vi "Liblinear - Scale Problem Linear.vi"(8 "error in (no error)":errorcluster, 10 "X Scaling limits":cluster{"X lower":dbl, "X upper":dbl}={"X lower"=0.0, "X upper"=1.0}, 11 "Problem":T1={"y"=[], "x"=[], "bias"=-1.0}) -> (0 "error out":errorcluster, 2 "xmaxmin":cluster{"min":dbl, "max":dbl}[](array[cluster]), 3 "Scaled problem":T1={"y"=[], "x"=[], "bias"=-1.0})   [LabVIEW 2015]
doc: "Scales the problem similarly to the svm-scale tool bundled with libsvm.\nAlways use the output from this VI to scale the test set instead of scaling individually."
uses:
  Liblinear/Controls/liblinear_problem.ctl
  LibSVM Sparse/Wrapper API/Controls/svm_node.ctl
  Controls/Statemachine_ScaleProblem.ctl
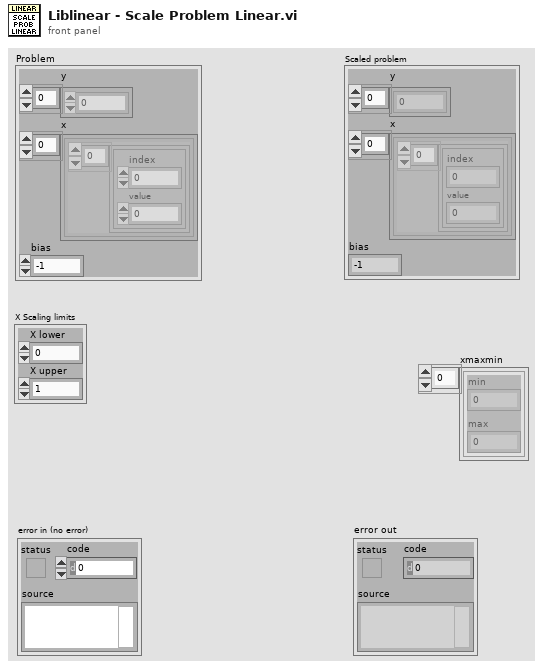
[diagram p1: front panel]
types:
  T1 = typedef "liblinear_problem.ctl" = cluster{"y":dbl[], "x":cluster{T2[]}[], "bias":dbl}
  T2 = typedef "svm_node.ctl" = cluster{"index":i32, "value":dbl}
  T3 = typedef "Statemachine_ScaleProblem.ctl" = enum16{"Input verification: Limits", "Input verification: Ascending indices", "Find max/min index", "Find max/min features", "Scale", "Stop"}
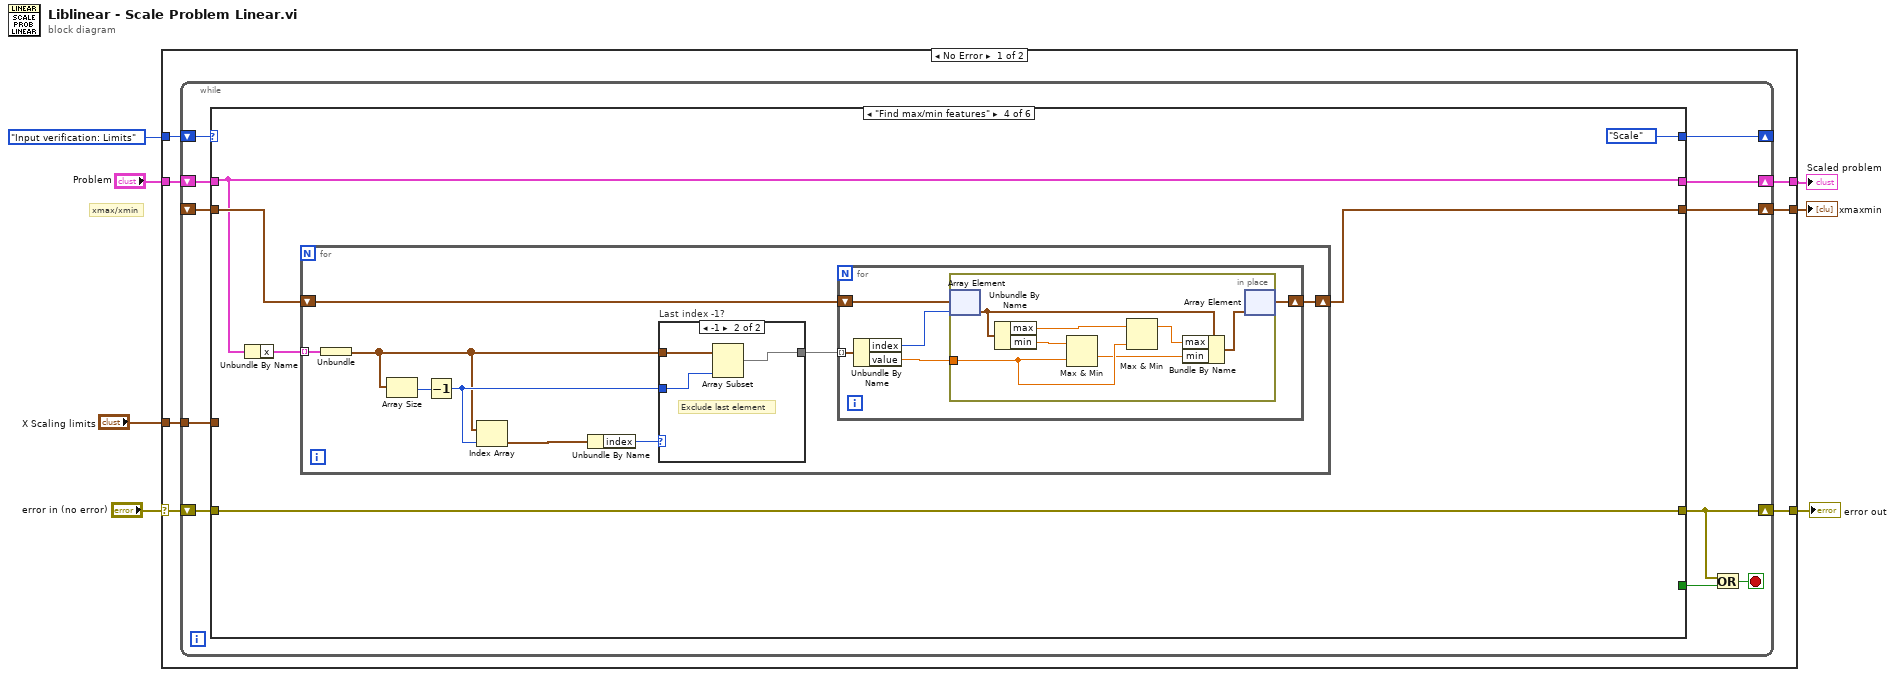
[diagram p0: block diagram]
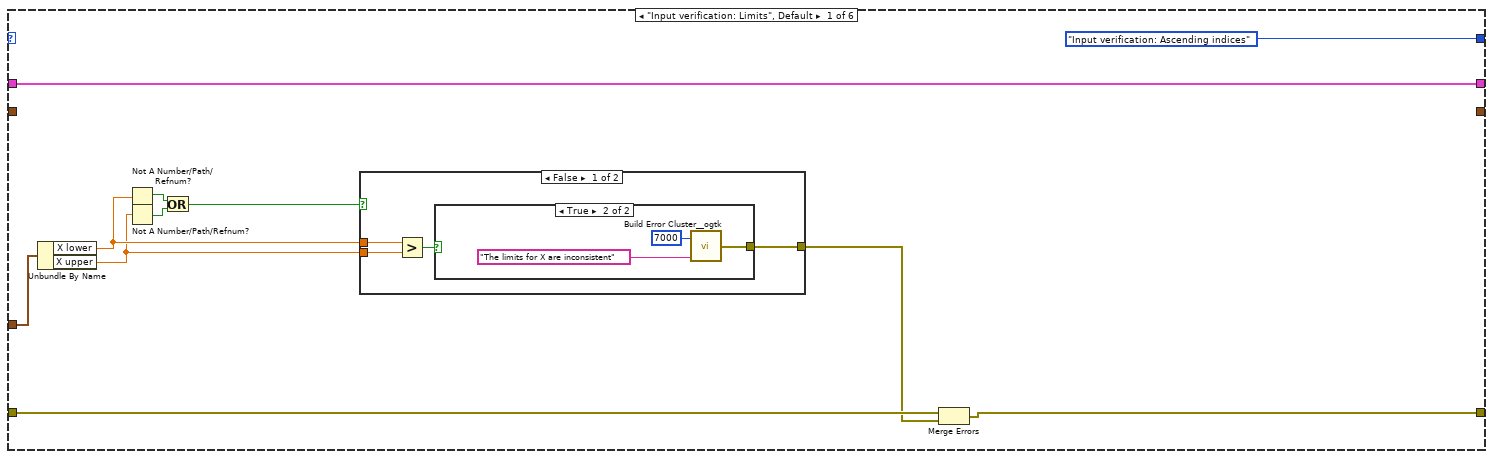
[diagram p2: hidden frame]
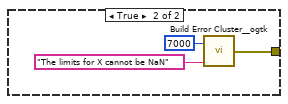
[diagram p4: hidden frame]
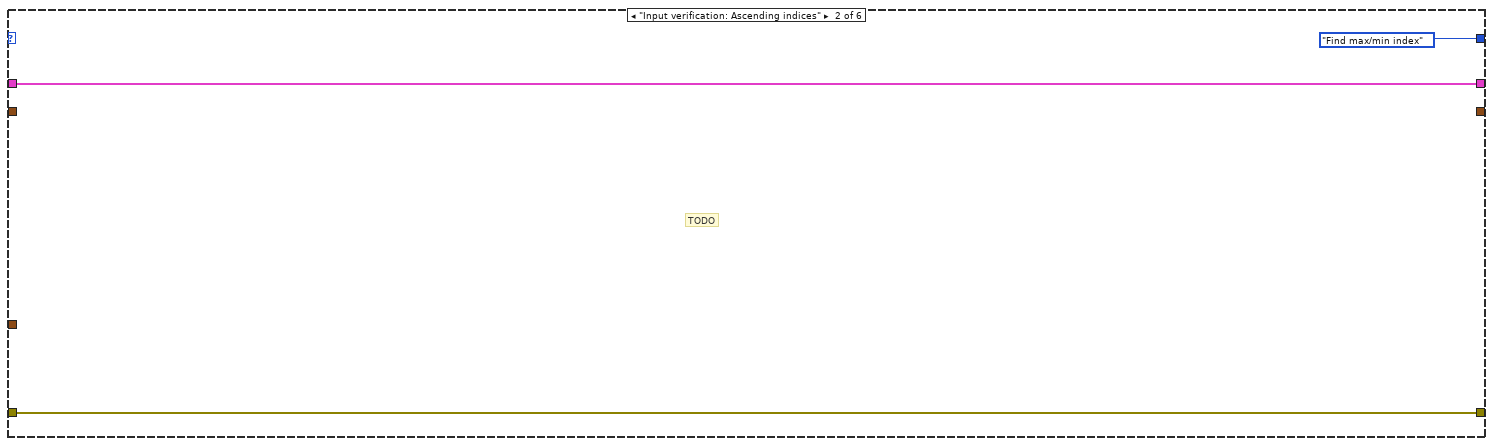
[diagram p5: hidden frame]
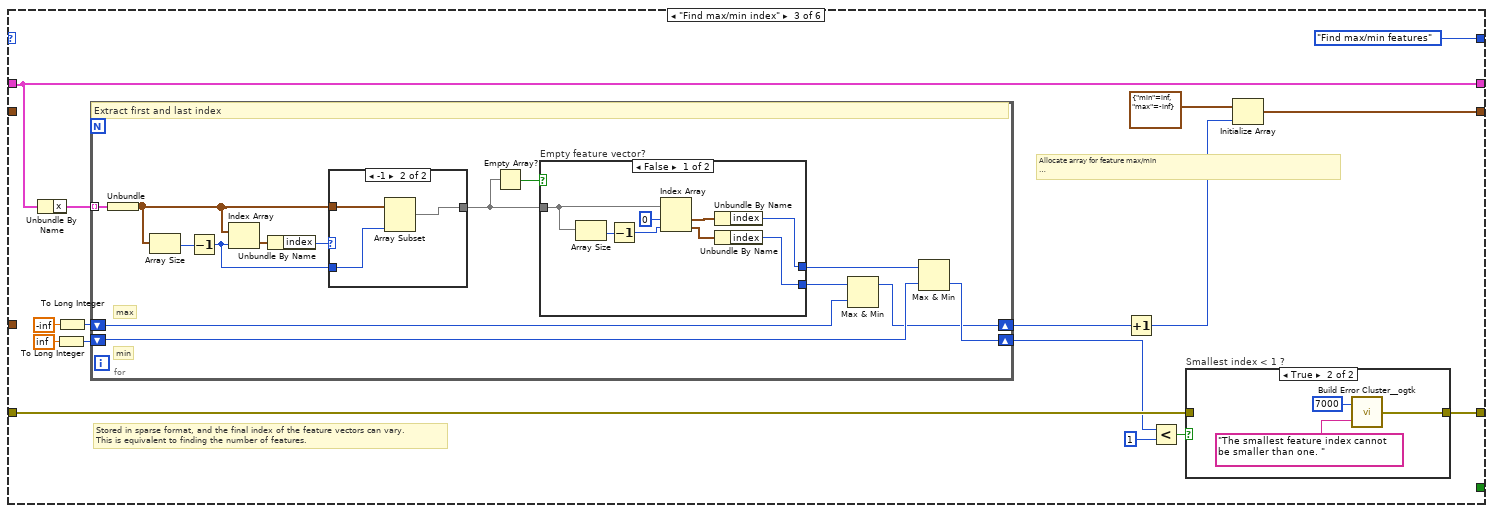
[diagram p6: hidden frame]
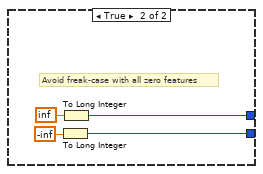
[diagram p9: hidden frame]
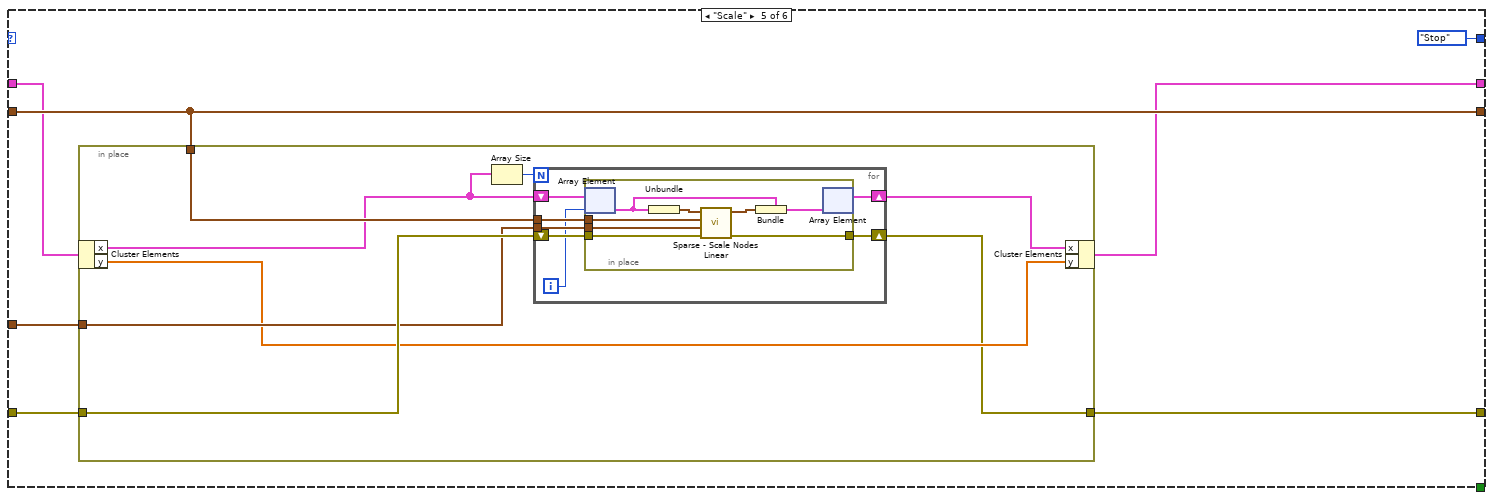
[diagram p11: hidden frame]
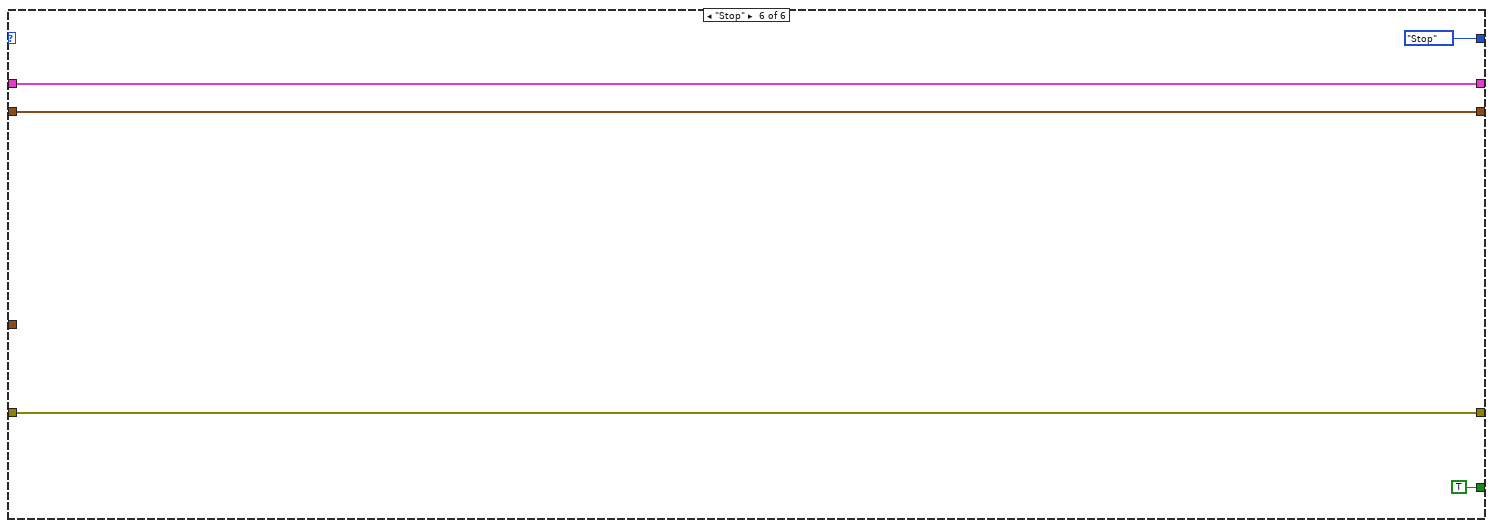
[diagram p12: hidden frame]
diagram:
  # "xmax/xmin"
  n1 = case shown="No Error" "error in (no error)" {
    selector: "error in (no error)" -> [w14 w166]
    tunnel: [w11 w166] -> w7
    tunnel: "Problem" -> [w8 _]
    tunnel: "X Scaling limits" -> [w12 _]
    tunnel: Statemachine_ScaleProblem."Input verification: Limits" ("Statemachine_ScaleProblem") -> [w13 _]
    tunnel: [w10 _] -> w3
    tunnel: [w9 _] -> w2
    frame No Error {
      n2 = while {
        shift-right: [w22] -> _
        shift-left: w13 -> [w25]
        tunnel: w12 -> [w24]
        shift-right: [w17] -> w11
        shift-left: w14 -> [w23]
        shift-right: [w21] -> w10
        shift-left: _ -> [w20]
        shift-right: [w19] -> w9
        shift-left: w8 -> [w18]
        stop <- w16 stop-if-true
        n3 = case shown="\"Find max/min features\"" w25 {
          tunnel: w24 -> [w36 _ _ _ w136 _]
          tunnel: w23 -> [w30 w49 w57 w102 w135 w164]
          tunnel: [w28 w49 w58 w102 w134 w164] -> w17
          tunnel: [Statemachine_ScaleProblem."Input verification: Ascending indices" ("Statemachine_ScaleProblem") Statemachine_ScaleProblem."Find max/min index" ("Statemachine_ScaleProblem") Statemachine_ScaleProblem."Find max/min features" ("Statemachine_ScaleProblem") Statemachine_ScaleProblem."Scale" ("Statemachine_ScaleProblem") Statemachine_ScaleProblem."Stop" ("Statemachine_ScaleProblem") Statemachine_ScaleProblem."Stop" ("Statemachine_ScaleProblem")] -> w22
          tunnel: [_ _ w54 w103 w133 w163] -> w21
          tunnel: w20 -> [_ _ _ w104 w133 w163]
          tunnel: [w26 w47 w52 w100 w131 w162] -> w19
          tunnel: w18 -> [w26 w47 w52 w100 w132 w162]
          tunnel: [_ _ _ _ _ TRUE] -> w15
          frame "Input verification: Limits", Default {
            n4 = Unbundle By Name(w36) -> ("X lower"=w32:dbl, "X upper"=w31:dbl)
            n5 = Not A Number/Path/Refnum?(number/path/refnum=w32) -> (NaN/Path/Refnum?=w34:bool)
            n6 = Not A Number/Path/Refnum?(number/path/refnum=w31) -> (NaN/Path/Refnum?=w35:bool)
            n7 = Or(x=w34, y=w35) -> (x .or. y?=w33:bool)
            n8 = case shown="False" w33 {
              tunnel: w32 -> [w39 _]
              tunnel: w31 -> [w38 _]
              tunnel: [w37 w44] -> w29
              frame False {
                n9 = Greater?(x=w39, y=w38) -> (0:w40:bool)
                n10 = case shown="True" w40 {
                  tunnel: [_ w41] -> w37
                  frame False {
                  }
                  frame True {
                    n11 = call <userlib>:"Build Error Cluster__ogtk.vi"("String to Prepend to source (\"\")"="The limits for X are inconsistent" ("String to Prepend to source (\"\")"), "code"=7000) -> ("error out"=w41:errorcluster)
                  }
                }
              }
              frame True {
                n12 = call <userlib>:"Build Error Cluster__ogtk.vi"("String to Prepend to source (\"\")"="The limits for X cannot be NaN" ("String to Prepend to source (\"\")"), "code"=7000) -> ("error out"=w44:errorcluster)
              }
            }
            n13 = Merge Errors(w30, w29) -> (w28:errorcluster)
          }
          frame "Input verification: Ascending indices" {
            # "TODO"
          }
          frame "Find max/min index" {
            # "Allocate array for feature max/min\n\n0th index is unused, avoids having to increment index all the time"
            # "Stored in sparse format, and the final index of the feature vectors can vary.\nThis is equivalent to finding the number of features."
            n14 = Unbundle By Name(w52) -> ("x"=w65:cluster{T2[]}[])
            n15 = To Long Integer(number=inf) -> (32bit integer=w63:i32)
            n16 = To Long Integer(number=-inf) -> (32bit integer=w61:i32)
            n17 = for {
              tunnel: w65 -> [w83] mode=indexing
              shift-right: [w77] -> w51
              shift-left: w61 -> [w81]
              shift-right: [w78] -> w55
              shift-left: w63 -> [w79]
              # "min"
              # "max"
              # "Extract first and last index"
              n18 = Unbundle(w83) -> (w72:T2[])
              n19 = Array Size(array=w72) -> (size(s)=w75:i32)
              n20 = Decrement(x=w75) -> (x-1=w71:i32)
              n21 = Index Array(array=w72, index=w71) -> (element=w74:T2)
              n22 = Unbundle By Name(w74) -> ("index"=w73:i32)
              n23 = case shown="-1" w73 {
                tunnel: w72 -> [w84 w87]
                tunnel: w71 -> [_ w86]
                tunnel: [w84 w85] -> w70
                frame Default {
                }
                frame -1 {
                  n24 = Array Subset(array=w87, length=w86) -> (w85:T2[])  [unwired: 1 in]
                }
              }
              n25 = Empty Array?(array=w70) -> (empty?=w82:bool)
              n26 = case "Empty feature vector?" shown="False" w82 {
                tunnel: [w88 w98] -> w76
                tunnel: [w93 w99] -> w80
                tunnel: w70 -> [w91 _]
                frame False {
                  n27 = Array Size(array=w91) -> (size(s)=w90:i32)
                  n28 = Decrement(x=w90) -> (x-1=w89:i32)
                  n29 = Index Array(array=w91, index #1=0 ("index"), index #2=w89) -> (element #1=w94:T2, element #2=w92:T2)
                  n30 = Unbundle By Name(w94) -> ("index"=w93:i32)
                  n31 = Unbundle By Name(w92) -> ("index"=w88:i32)
                }
                frame True {
                  # "Avoid freak-case with all zero features"
                  n32 = To Long Integer(number=-inf) -> (32bit integer=w98:i32)
                  n33 = To Long Integer(number=inf) -> (32bit integer=w99:i32)
                }
              }
              n34 = Max & Min(x=w76, y=w81) -> (max(x,y)=w77:i32)  [unwired: 1 out]
              n35 = Max & Min(x=w80, y=w79) -> (min(x,y)=w78:i32)  [unwired: 1 out]
            }
            n36 = Increment(x=w51) -> (x+1=w50:i32)
            n37 = Less?(x=w55, y=1) -> (x < y?=w59:bool)
            n38 = case "Smallest index < 1 ?" shown="True" w59 {
              tunnel: [w66 w69] -> w58
              tunnel: w57 -> [w66 _]
              frame False {
              }
              frame True {
                n39 = call <userlib>:"Build Error Cluster__ogtk.vi"("String to Prepend to source (\"\")"="The smallest feature index cannot be smaller than one. " ("String to Prepend to source (\"\")"), "code"=7000) -> ("error out"=w69:errorcluster)
              }
            }
            n40 = Initialize Array(cluster{"min":dbl, "max":dbl} {"min"=inf, "max"=-inf}, w50) -> (w54:cluster{"min":dbl, "max":dbl}[])
          }
          frame "Find max/min features" {
            n41 = Unbundle By Name(w100) -> ("x"=w105:cluster{T2[]}[])
            n42 = for {
              tunnel: w105 -> [w114] mode=indexing
              shift-right: [w107] -> w103
              shift-left: w104 -> [w113]
              n43 = Unbundle(w114) -> (w106:T2[])
              n44 = Array Size(array=w106) -> (size(s)=w112:i32)
              n45 = Decrement(x=w112) -> (x-1=w109:i32)
              n46 = Index Array(array=w106, index=w109) -> (element=w111:T2)
              n47 = Unbundle By Name(w111) -> ("index"=w110:i32)
              n48 = case "Last index -1?" shown="-1" w110 {
                tunnel: w106 -> [w115 w118]
                tunnel: w109 -> [_ w117]
                tunnel: [w115 w116] -> w108
                frame Default {
                }
                frame -1 {
                  # "Exclude last element"
                  n49 = Array Subset(array=w118, length=w117) -> (w116:T2[])  [unwired: 1 in]
                }
              }
              n50 = for {
                tunnel: w108 -> [w123] mode=indexing
                shift-right: [w119] -> w107
                shift-left: w113 -> [w122]
                n51 = Unbundle By Name(w123) -> ("index"=w121:i32, "value"=w120:dbl)
                n52 = in-place {
                  in-place-border: w120 -> [w128]
                  n53 = in-place-array #1(w122, w121) -> (w127:cluster{"min":dbl, "max":dbl})
                  n54 = Unbundle By Name(w127) -> ("max"=w129:dbl, "min"=w130:dbl)
                  n55 = Max & Min(x=w130, y=w128) -> (min(x,y)=w125:dbl)  [unwired: 1 out]
                  n56 = Max & Min(x=w129, y=w128) -> (max(x,y)=w124:dbl)  [unwired: 1 out]
                  n57 = Bundle By Name(cluster=w127, "max"=w124, "min"=w125) -> (w126:cluster{"min":dbl, "max":dbl})
                  n58 = in-place-array #1(w126) -> (w119:cluster{"min":dbl, "max":dbl}[])  [unwired: 1 out]
                }
              }
            }
          }
          frame "Scale" {
            n59 = in-place {
              in-place-border: w136 -> [w140]
              in-place-border: w135 -> [w145]
              in-place-border: [w138] -> w134
              in-place-border: w133 -> [w144]
              n60 = in-place-cluster #2(w132) -> ("x"=w142:cluster{T2[]}[], "y"=w139:dbl[])
              n61 = Array Size(array=w142) -> (size(s)=w143:i32)
              n62 = for {
                N: w143 -> [_]
                tunnel: w144 -> [w151]
                shift-right: [w150] -> w138
                shift-left: w145 -> [w152]
                tunnel: w140 -> [w149]
                shift-right: [w146] -> w141
                shift-left: w142 -> [w148]
                i -> [w147]
                n63 = in-place {
                  in-place-border: w152 -> [w159]
                  in-place-border: w151 -> [w160]
                  in-place-border: [w158] -> w150
                  in-place-border: w149 -> [w153]
                  n64 = in-place-array #3(w148, w147) -> (w154:cluster{T2[]})
                  n65 = Unbundle(w154) -> (w157:T2[])
                  n66 = call "Sparse - Scale Nodes Linear.vi"("error in (no error)"=w159, "Scaling limits"=w153, "xmaxmin"=w160, "x"=w157) -> ("error out"=w158:errorcluster, "x scaled"=w156:T2[])  [unwired: 6 in]
                  n67 = Bundle(cluster=w154, w156) -> (w155:cluster{T2[]})
                  n68 = in-place-array #3(w155) -> (w146:cluster{T2[]}[])  [unwired: 1 out]
                }
              }
              n69 = in-place-cluster #2("x"=w141, "y"=w139) -> (w131:T1)
            }
          }
          frame "Stop" {
          }
        }
        n70 = Or(x=w17, y=w15) -> (x .or. y?=w16:bool)
      }
    }
    frame Error {
    }
  }
  "error out" <- w7
  "xmaxmin" <- w3
  "Scaled problem" <- w2
